vi "task.vi"(8 "error in (no error)":errorcluster, 10 "taskChannel":refnum<class "ITaskChannel.lvclass">, 11 "ITask in":refnum<class "ITask.lvclass">) -> (0 "error out":errorcluster, 3 "ITask out":refnum<class "ITask.lvclass">)   [LabVIEW 2023, in "TaskMock.lvclass"]
uses:
  TaskMock.lvclass
  source/ITask/ITask.lvclass
  source/ITaskChannel/ITaskChannel.lvclass
  source/BoolNotifierTaskChannel/BoolNotifierTaskChannel.lvclass
  source/BoolNotifierTaskChannel/BoolNotifierTaskChannel.lvclass/BoolNotifierTaskChannel.ctl
  TaskMock.lvclass/TaskMock.ctl
  source/BoolNotifierTaskChannel/Read notifierRef.vi
panel:
  out "i_loop":i32
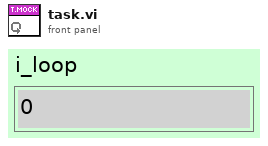
[diagram p1: front panel]
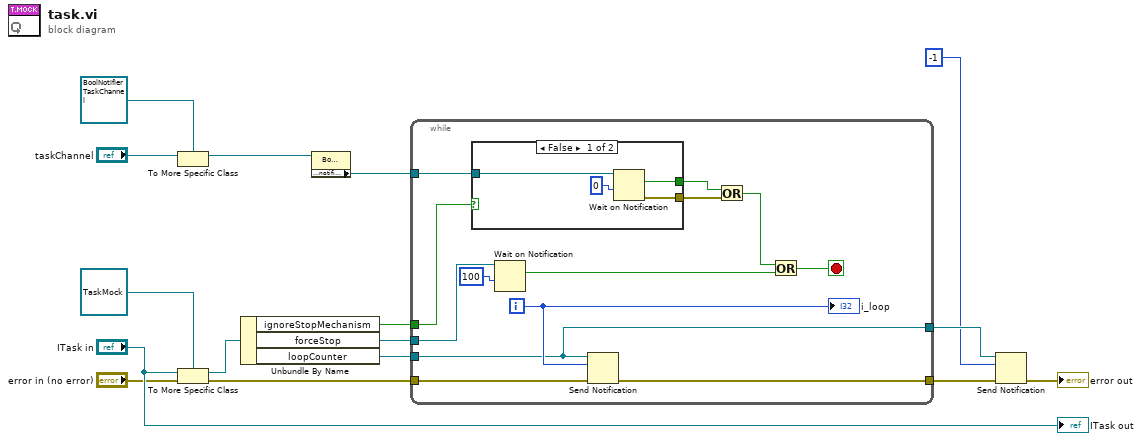
[diagram p0: block diagram]
diagram:
  n1 = To More Specific Class(target class=refnum<class "BoolNotifierTaskChannel.lvclass"> refnum ("TLC_Daemon.lvlib:NotifierStopMechanism.lvclass"), reference="taskChannel") -> (specific class reference=w3:refnum<class "BoolNotifierTaskChannel.lvclass">)  [unwired: 1 in, 1 out]
  n2 = To More Specific Class(target class=refnum<class "TaskMock.lvclass"> refnum ("TaskMock.lvclass"), reference="ITask in", error in="error in (no error)") -> (specific class reference=w14:refnum<class "TaskMock.lvclass">, error out=w12:errorcluster)
  n3 = Unbundle By Name(w14) -> ("ignoreStopMechanism"=w1:bool, "forceStop"=w10:refnum<notifier>, "loopCounter"=w13:refnum<notifier>)
  n4 = property class="BoolNotifierTaskChannel.lvclass"(reference=w3) -> ("Properties:notifierRef"=w2:refnum<notifier>)  [unwired: 1 in, 2 out]
  n5 = while {
    tunnel: w2 -> [w29]
    tunnel: w13 -> [w18]
    tunnel: w12 -> [w27]
    tunnel: [w26] -> w7
    tunnel: w10 -> [w22]
    tunnel: [w18] -> w9
    tunnel: w1 -> [w17]
    i -> [w28]
    stop <- w19 stop-if-true
    n6 = case shown="False" w17 {
      tunnel: w29 -> [w33 _]
      tunnel: [w31 _] -> w25
      tunnel: [w30 _] -> w24
      frame False {
        n7 = Wait on Notification(notifier=w33, timeout in ms (-1)=0) -> (notification=w30:bool, error out=w31:errorcluster)  [unwired: 2 in, 2 out]
      }
      frame True {
      }
    }
    n8 = Wait on Notification(notifier=w22, timeout in ms (-1)=100) -> (notification=w21:bool)  [unwired: 2 in, 3 out]
    n9 = Send Notification(notification=w28, notifier=w18, error in (no error)=w27) -> (error out=w26:errorcluster)  [unwired: 1 out]
    n10 = Or(x=w24, y=w25) -> (x .or. y?=w20:bool)
    n11 = Or(x=w20, y=w21) -> (x .or. y?=w19:bool)
    "i_loop" <- w28
  }
  n12 = Send Notification(notification=-1, notifier=w9, error in (no error)=w7) -> (error out=→"error out":errorcluster)  [unwired: 1 out]
  "ITask out" <- "ITask in"
